vi "test Compare Parameters.vi"(8 "error in":errorcluster, 11 "TestCase in":refnum<class "Refresh.lvclass">) -> (0 "error out":errorcluster, 3 "TestCase out":refnum<class "Refresh.lvclass">)   [LabVIEW 2020, in "Refresh.lvclass"]
uses:
  Refresh.lvclass
  <vilib>/addons/_JKI Toolkits/VI Tester/TestCase.llb/TestCase.lvclass
  System Explorer/Implementation/Implementation.lvlib
  Encoding and Decoding/Encoding.ctl
  Encoding and Decoding/Encoding and Decoding.lvlib
  Shared/Parameter Definition.ctl
  Shared/VS Channel Definition for Parameter.ctl
  System Explorer/Implementation/System Explorer/Types/Refresh Symbols.ctl
  System Explorer/Implementation/System Explorer/Types/Refresh Listbox.ctl
  C:/Program Files (x86)/National Instruments/LabVIEW 2020/vi.lib/addons/_JKI Toolkits/VI Tester/TestCase.llb/TestCase.lvclass
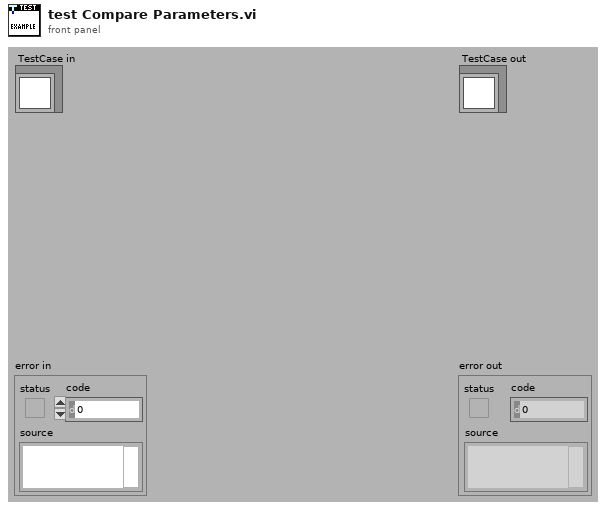
[diagram p1: front panel]
types:
  T1 = typedef "VS Channel Definition for Parameter.ctl" = cluster{"name":string, "default value":dbl, "unit":string, "Parameter":T2}
  T2 = typedef "Parameter Definition.ctl" = cluster{"start index":i32, "size":i32, "encoding":T3, "signed":bool, "scale multiplier":dbl, "scale offset":dbl}
  T3 = typedef "Encoding and Decoding.lvlib/Encoding.ctl" = enum16{"BNR", "BCD", "Discrete"}
  T4 = typedef "Ballard ARINC 429 System Explorer.lvlib/Implementation.lvlib/Refresh Listbox.ctl" = cluster{"Item Names":string[], "Item Symbol":T5, "Change Flag":bool}
  T5 = typedef "Ballard ARINC 429 System Explorer.lvlib/Implementation.lvlib/Refresh Symbols.ctl" = enum16{"Blank", "Port", "Incoming", "Outgoing", "Label", "Word", "Parameter", "ARINC-429", "Config Files", "Channel Spec", "Item"}
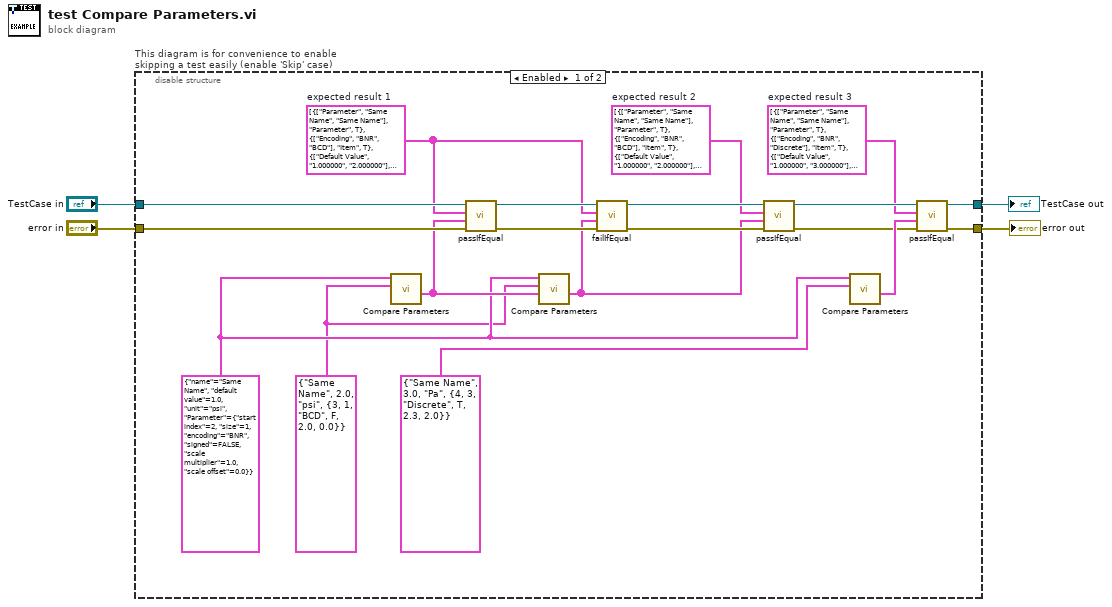
[diagram p0: block diagram]
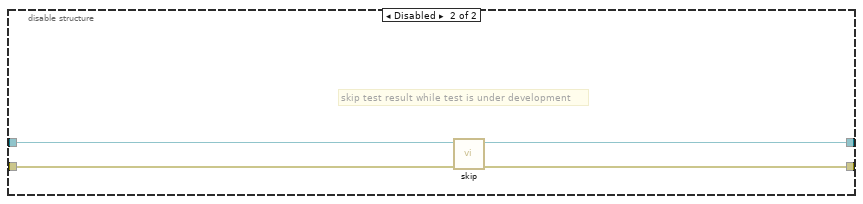
[diagram p2: hidden frame]
diagram:
  n1 = disable-structure "This diagram is for convenience to enable skipping a test easily (enable 'Skip' case)" shown="Enabled" {
    disable-tunnel: "TestCase in" -> [w23 w27]
    disable-tunnel: [w11 w25] -> w1
    disable-tunnel: [w13 w26] -> w3
    disable-tunnel: "error in" -> [w22 w24]
    frame Enabled {
      w5 = T4[] [{"Item Names"=["Parameter", "Same Name", "Same Name"], "Item Symbol"=enum."Parameter", "Change Flag"=TRUE}, {"Item Names"=["Encoding", "BNR", "Discrete"], "Item Symbol"=enum."Item", "Change Flag"=TRUE}, {"Item Names"=["Default Value", "1.000000", "3.000000"], "Item Symbol"=enum."Item", "Change Flag"=TRUE}, {"Item Names"=["Start Index", "2", "4"], "Item Symbol"=enum."Item", "Change Flag"=TRUE}, {"Item Names"=["Size", "1", "3"], "Item Symbol"=enum."Item", "Change Flag"=TRUE}, {"Item Names"=["Signed", "FALSE", "TRUE"], "Item Symbol"=enum."Item", "Change Flag"=TRUE}, {"Item Names"=["Scale Factor", "1.000000", "2.300000"], "Item Symbol"=enum."Item", "Change Flag"=TRUE}, {"Item Names"=["Scale Offset", "0.000000", "2.000000"], "Item Symbol"=enum."Item", "Change Flag"=TRUE}, {"Item Names"=["Unit", "psi", "Pa"], "Item Symbol"=enum."Item", "Change Flag"=TRUE}]  # expected result 3
      w6 = T4[] [{"Item Names"=["Parameter", "Same Name", "Same Name"], "Item Symbol"=enum."Parameter", "Change Flag"=TRUE}, {"Item Names"=["Encoding", "BNR", "BCD"], "Item Symbol"=enum."Item", "Change Flag"=TRUE}, {"Item Names"=["Default Value", "1.000000", "2.000000"], "Item Symbol"=enum."Item", "Change Flag"=TRUE}, {"Item Names"=["Start Index", "2", "3"], "Item Symbol"=enum."Item", "Change Flag"=TRUE}, {"Item Names"=["Size", "1", "1"], "Item Symbol"=enum."Item", "Change Flag"=FALSE}, {"Item Names"=["Signed", "FALSE", "FALSE"], "Item Symbol"=enum."Item", "Change Flag"=FALSE}, {"Item Names"=["Scale Factor", "1.000000", "2.000000"], "Item Symbol"=enum."Item", "Change Flag"=TRUE}, {"Item Names"=["Scale Offset", "0.000000", "0.000000"], "Item Symbol"=enum."Item", "Change Flag"=FALSE}, {"Item Names"=["Unit", "psi", "psi"], "Item Symbol"=enum."Item", "Change Flag"=FALSE}, {"Item Names"=["Parameter", "Same Name", "Same Name"], "Item Symbol"=enum."Parameter", "Change Flag"=TRUE}, {"Item Names"=["Encoding", "BNR", "BCD"], "Item Symbol"=enum."Item", "Change Flag"=TRUE}, {"Item Names"=["Default Value", "1.000000", "2.000000"], "Item Symbol"=enum."Item", "Change Flag"=TRUE}, {"Item Names"=["Start Index", "2", "3"], "Item Symbol"=enum."Item", "Change Flag"=TRUE}, {"Item Names"=["Size", "1", "1"], "Item Symbol"=enum."Item", "Change Flag"=FALSE}, {"Item Names"=["Signed", "FALSE", "FALSE"], "Item Symbol"=enum."Item", "Change Flag"=FALSE}, {"Item Names"=["Scale Factor", "1.000000", "2.000000"], "Item Symbol"=enum."Item", "Change Flag"=TRUE}, {"Item Names"=["Scale Offset", "0.000000", "0.000000"], "Item Symbol"=enum."Item", "Change Flag"=FALSE}, {"Item Names"=["Unit", "psi", "psi"], "Item Symbol"=enum."Item", "Change Flag"=FALSE}]  # expected result 2
      w9 = T4[] [{"Item Names"=["Parameter", "Same Name", "Same Name"], "Item Symbol"=enum."Parameter", "Change Flag"=TRUE}, {"Item Names"=["Encoding", "BNR", "BCD"], "Item Symbol"=enum."Item", "Change Flag"=TRUE}, {"Item Names"=["Default Value", "1.000000", "2.000000"], "Item Symbol"=enum."Item", "Change Flag"=TRUE}, {"Item Names"=["Start Index", "2", "3"], "Item Symbol"=enum."Item", "Change Flag"=TRUE}, {"Item Names"=["Size", "1", "1"], "Item Symbol"=enum."Item", "Change Flag"=FALSE}, {"Item Names"=["Signed", "FALSE", "FALSE"], "Item Symbol"=enum."Item", "Change Flag"=FALSE}, {"Item Names"=["Scale Factor", "1.000000", "2.000000"], "Item Symbol"=enum."Item", "Change Flag"=TRUE}, {"Item Names"=["Scale Offset", "0.000000", "0.000000"], "Item Symbol"=enum."Item", "Change Flag"=FALSE}, {"Item Names"=["Unit", "psi", "psi"], "Item Symbol"=enum."Item", "Change Flag"=FALSE}]  # expected result 1
      w16 = T1 {"name"="Same Name", "default value"=1.0, "unit"="psi", "Parameter"={"start index"=2, "size"=1, "encoding"=enum."BNR", "signed"=FALSE, "scale multiplier"=1.0, "scale offset"=0.0}} ("old parameter")
      w7 = T1 {"name"="Same Name", "default value"=2.0, "unit"="psi", "Parameter"={"start index"=3, "size"=1, "encoding"=enum."BCD", "signed"=FALSE, "scale multiplier"=2.0, "scale offset"=0.0}} ("new parameter")
      n2 = call "Compare Parameters.vi"("new parameter"=w7, "old parameter"=w16) -> ("refresh listbox out"=w21:T4[])  [unwired: 8 in, 1 out]
      n3 = call-dynamic "passIfEqual.vi"("error in (no error)"=w22, "y"=w21, "x"=w9, "TestCase in"=w23) -> ("error out"=w20:errorcluster, "TestCase out"=w10:refnum<class "Refresh.lvclass">)  [unwired: 6 in]
      n4 = call "Compare Parameters.vi"("refresh listbox"=w21, "new parameter"=w7, "old parameter"=w16) -> ("refresh listbox out"=w17:T4[])  [unwired: 7 in, 1 out]
      n5 = call-dynamic "failIfEqual.vi"("error in (no error)"=w20, "y"=w17, "x"=w9, "TestCase in"=w10) -> ("error out"=w19:errorcluster, "TestCase out"=w18:refnum<class "Refresh.lvclass">)  [unwired: 6 in]
      n6 = call-dynamic "passIfEqual.vi"("error in (no error)"=w19, "y"=w17, "x"=w6, "TestCase in"=w18) -> ("error out"=w14:errorcluster, "TestCase out"=w12:refnum<class "Refresh.lvclass">)  [unwired: 6 in]
      n7 = call "Compare Parameters.vi"("new parameter"=T1 {"name"="Same Name", "default value"=3.0, "unit"="Pa", "Parameter"={"start index"=4, "size"=3, "encoding"=enum."Discrete", "signed"=TRUE, "scale multiplier"=2.3, "scale offset"=2.0}}, "old parameter"=w16) -> ("refresh listbox out"=w15:T4[])  [unwired: 8 in, 1 out]
      n8 = call-dynamic "passIfEqual.vi"("error in (no error)"=w14, "y"=w15, "x"=w5, "TestCase in"=w12) -> ("error out"=w13:errorcluster, "TestCase out"=w11:refnum<class "Refresh.lvclass">)  [unwired: 6 in]
    }
    frame Disabled {
      # "skip test result while test is under development"
      n9 = call <vilib>:"skip.vi"("error in (no error)"=w24, "TestCase in"=w27) -> ("error out"=w26:errorcluster, "TestCase out"=w25:refnum<class "Refresh.lvclass">)  [unwired: 8 in]
    }
  }
  "error out" <- w3
  "TestCase out" <- w1
